vi "DllFxpIntAccumulator_Fxp.vi"(6 "enable":bool, 8 "cinNbin":bool, 9 "isSub":bool, 10 "load":bool, 11 "x":fxp<+,16,16>) -> (2 "coutNbout":bool, 3 "sum":fxp<+,32,32>)   [LabVIEW 2017]
uses:
  <vilib>/rvi/FXPMathLib/basic elements/FxpIntAccumulator/subVIs/nifxpmath_IntAccumulator_SimConfig.ctl
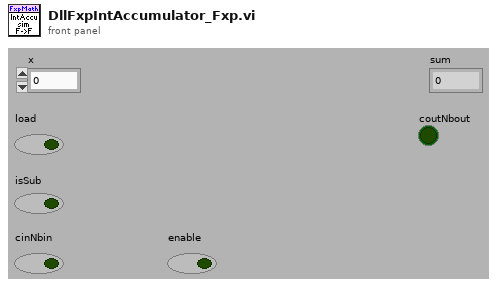
[diagram p1: front panel]
types:
  T1 = typedef "nifxpmath_IntAccumulator_SimConfig.ctl" = cluster{"kWordLengthIn":u16, "kWordLengthOut":u16, "kPrescaling":u16, "kNumOfCh":u16, "kIsSigned":bool, "kIsRegOut":bool}
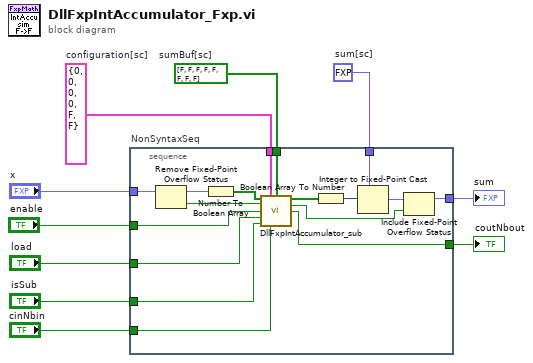
[diagram p0: block diagram]
diagram:
  w1 = T1 {"kWordLengthIn"=0, "kWordLengthOut"=0, "kPrescaling"=0, "kNumOfCh"=0, "kIsSigned"=FALSE, "kIsRegOut"=FALSE}  # configuration[sc]
  w5 = fxp<+,32,32> 0.0  # sum[sc]
  w3 = bool[] [FALSE, FALSE, FALSE, FALSE, FALSE, FALSE, FALSE, FALSE]  # sumBuf[sc]
  n1 = stacked-sequence "NonSyntaxSeq" {
    tunnel: [w24] -> w9
    tunnel: "load" -> [w19]
    tunnel: "enable" -> [w20]
    tunnel: w1 -> [w23]
    tunnel: "cinNbin" -> [w17]
    tunnel: "isSub" -> [w18]
    tunnel: "x" -> [w27]
    tunnel: w5 -> [w11]
    tunnel: [w25] -> w4
    tunnel: w3 -> [w22]
    frame #0 {
      n2 = Remove Fixed-Point Overflow Status(3:w27) -> (0:w15:bool, 1:w26:fxp<+,16,16>)
      n3 = Number To Boolean Array(number=w26) -> (Boolean array=w21:bool[])
      n4 = call <vilib>:"DllFxpIntAccumulator_sub.vi"("x"=w21, "configuration[sc]"=w23, "sumBuf[sc]"=w22, "xov"=w15, "enable"=w20, "load"=w19, "isSub"=w18, "cinNbin"=w17) -> ("s"=w16:bool[], "sov"=w14:bool, "coutNbout"=w24:bool)  [unwired: 5 out]
      n5 = Boolean Array To Number(Boolean array=w16) -> (number=w13:u64)
      n6 = Integer to Fixed-Point Cast(fixed-point type=w11, integer=w13) -> (fixed-point=w12:fxp<+,32,32>)
      n7 = Include Fixed-Point Overflow Status(2:w14, 3:w12) -> (1:w25:fxp<+,32,32>)
    }
  }
  "coutNbout" <- w9
  "sum" <- w4
